vi "Init.vi"(8 "error in (no error)":errorcluster, 11 "Event_TextLog in":refnum<class "Event_TextLog.lvclass">) -> (0 "error out":errorcluster, 3 "Event_TextLog out":refnum<class "Event_TextLog.lvclass">)   [LabVIEW 2021, in "Event_TextLog.lvclass"]
uses:
  Event_TextLog.lvclass
  Event_TextLog.lvclass/Event_TextLog.ctl
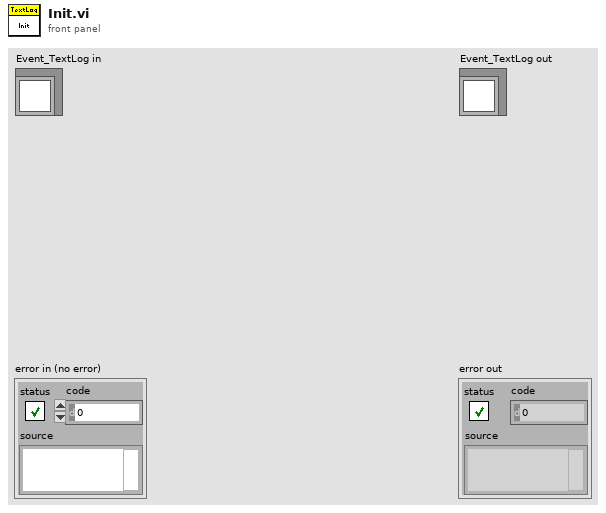
[diagram p1: front panel]
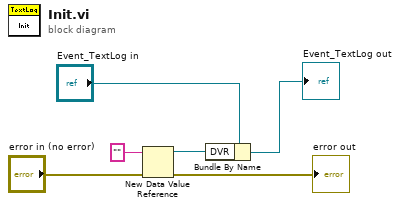
[diagram p0: block diagram]
diagram:
  n1 = New Data Value Reference(data value="", error in="error in (no error)") -> (data value reference=w2:refnum<data-value>, error out=→"error out":errorcluster)
  n2 = Bundle By Name(cluster="Event_TextLog in", "DVR"=w2) -> (→"Event_TextLog out":refnum<class "Event_TextLog.lvclass">)
